vi "Error Query (Multiple).vi"(0 "VISA resource name":refnum<visa-resource-name>, 5 "error in (no error)":errorcluster) -> (14 "VISA resource name out":refnum<visa-resource-name>, 17 "Error":i32[](array[numeric]), 18 "Error Message":string, 19 "error out":errorcluster)   [LabVIEW 2016, in "Keithley 2000.lvlib"]
doc: "This VI reads the error queue from the instrument. It expects to see errors in SCPI format (#,\"error message\"). It continues to read from the error queue until it reads a 0, \"No error\". If the instrument does not support an error query, a warning is returned."
uses:
  Keithley 2000.lvlib
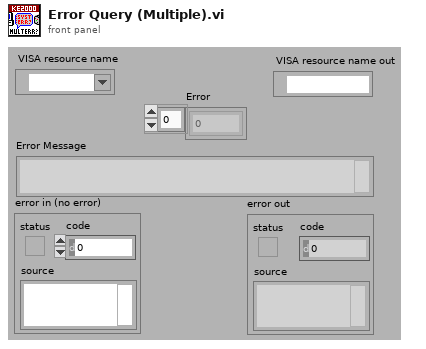
[diagram p1: front panel]
types:
  T1 = cluster{"Status":bool, "Error":i32, "source":string}
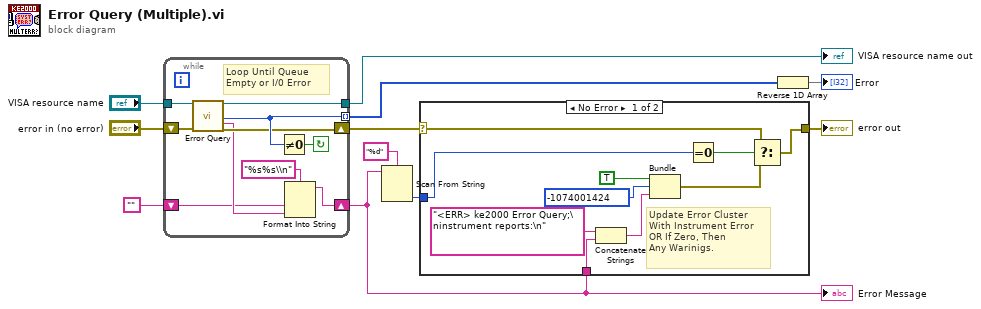
[diagram p0: block diagram]
diagram:
  n1 = while {
    tunnel: [w19] -> w9 mode=indexing
    shift-left: "" ("Empty String Constant") -> [w14]
    shift-right: [w12] -> w3
    tunnel: "VISA resource name" -> [w18]
    tunnel: [w21] -> w7
    shift-right: [w16] -> w5
    shift-left: "error in (no error)" -> [w17]
    stop <- w20 continue-if-true
    # "Loop Until Queue Empty or I/0 Error"
    n2 = call "Error Query.vi"("VISA resource name"=w18, "error in (no error)"=w17) -> ("VISA resource name out"=w21:refnum<visa-resource-name>, "Error"=w19:i32, "Error Message"=w15:string, "error out"=w16:errorcluster)  [unwired: 14 in]
    n3 = Not Equal To 0?(x=w19) -> (x != 0?=w20:bool)
    n4 = Format Into String(format string="%s%s\\n", w14, w15) -> (resulting string=w12:string)  [unwired: 2 in, 1 out]
  }
  "Error Message" <- w3
  "VISA resource name out" <- w7
  n5 = Scan From String(format string="%d", input string=w3) -> (output 1=w1:i32)  [unwired: 3 in, 3 out]
  n6 = case shown="No Error" w5 {
    selector: w5 -> [w22 w32]
    tunnel: w1 -> [w23 _]
    tunnel: [w25 w32] -> w10
    tunnel: w3 -> [w31 _]
    frame No Error {
      # "Update Error Cluster\nWith Instrument Error \nOR If Zero, Then \nAny Warinigs."
      n7 = Concatenate Strings("<ERR> ke2000 Error Query;\ninstrument reports:\n" ("Source"), w31) -> (w28:string)
      n8 = Bundle("Status"=TRUE, "Error"=-1074001424, w28) -> (w24:cluster{"Status":bool, "Error":i32, string})  [unwired: 1 in]
      n9 = Equal To 0?(x=w23) -> (x = 0?=w26:bool)
      n10 = Select(t=w22, s=w26, f=w24) -> (s? t:f=w25:T1)
    }
    frame Error {
      # "IO Error"
    }
  }
  "error out" <- w10
  n11 = Reverse 1D Array(array=w9) -> (reversed array=→"Error":i32[])
